vi "HFRR ADV v05 new software.vi"() -> ()   [LabVIEW 2025] (continued)
                "state1" <- w4567
              }
              frame Enabled {
              }
            }
            n3613 = stacked-sequence {
              tunnel: w4484 -> [w4592 _ _]
              tunnel: [_ _ w4608] -> _
              frame #0 {
                (unwired) FALSE ("convert eol (F)")
                w4594 = enum16{"start", "end", "current"}."start" ("pos mode (0:2)")
                n3614 = local read "Path"() -> (w4588:path)
                n3615 = Path To String(path=w4588) -> (string=w4600:string)
                n3616 = Concatenate Strings(w4600, "\\", "Sensor File Name") -> (w4601:string)
                n3617 = local write "standard output 2"(" ") -> ()
                n3618 = String To Path(string=w4601) -> (path=w4591:path)
                n3619 = call <vilib>:"Open_Create_Replace File.vi"("advisory dialog? (display:T)"=FALSE, "function (open:0)"=T25."create or replace", "file path"=w4591) -> ("error out"=w4604:errorcluster, "refnum"=w4603:refnum<file>)  [unwired: 5 in, 2 out]
                n3620 = Set File Position(refnum=w4603, from (0:start)=w4594, error in=w4604) -> (refnum out=w4584:refnum<file>, error out=w4583:errorcluster)  [unwired: 1 in]
                n3621 = Write to Binary File(file (use dialog)=w4584, data=" ", error in=w4583, 5:FALSE ("prepend array or string size? (T)")) -> (refnum out=w4595:refnum<file>, error out=w4596:errorcluster)  [unwired: 2 in, 1 out]
                n3622 = Set File Position(offset (in bytes) (0)=w4594, refnum=w4595, error in=w4596) -> (refnum out=w4587:refnum<file>, error out=w4586:errorcluster)  [unwired: 1 in]
                n3623 = Write to Binary File(file (use dialog)=w4587, data=w4592, error in=w4586, 5:FALSE ("prepend array or string size? (T)")) -> (error out=w4590:errorcluster)  [unwired: 2 in, 2 out]
                n3624 = flat-sequence {
                  tunnel: w4591 -> [w4606]
                  tunnel: w4590 -> [_]
                  frame #0 {
                    n3625 = call <vilib>:"Read Characters From File.vi"("file path (dialog if empty)"=w4606) -> ("character string"=→"Sensor Health JSON string":string)  [unwired: 5 in, 3 out]
                  }
                }
                "SinglePoint  2" <- w4592
              }
              frame #1 {
              }
              frame #2 {
                (unwired) "\"Stored\": true" ("string")
                n3626 = call <vilib>:"System Exec.vi"("run minimized? (F)"=TRUE, "wait until completion? (T)"=TRUE, "working directory"=path "C:/LAB-IQ-NXT", "command line"="C:\\LAB-IQ-NXT\\JPostH.bat") -> ("standard error"=→"Respose From Server 2":string, "standard output"=w4611:string)  [unwired: 4 in, 2 out]
                "standard output 2" <- w4611
                n3627 = Match Pattern(string=w4611, regular expression="JSONH Check String") -> (match substring=w4609:string, offset past match=w4608:i32)  [unwired: 1 in, 2 out]
                n3628 = Equal?(x=w4609, y="JSONH Check String") -> (x = y?=→"Upload \nConfirmed 2":bool)
              }
            }
            n3629 = Divide(x=w4451, y=3600.0 ("f")) -> (x/y=w4444:dbl)
            n3630 = local read "run time"() -> (w4501:string[])
            n3631 = Round To Nearest(number=w4444) -> (nearest integer value=w4443:dbl)
            n3632 = Number To Decimal String(number=w4443) -> (decimal integer string=w4442:string)  [unwired: 1 in]
            n3633 = Index Array(array="Sensor Information", index (col) #1=0 ("disabled index (col)"), index (col) #2=1 ("index (col)"), index (col) #3=2 ("index (col)"), index (col) #4=3 ("index (col)")) -> (element #1=→"Sensor name":string[], element #2=→"model num":string[], element #3=→"run time":string[], element #4=→"state":string[])  [unwired: 4 in]
            n3634 = Insert Into Array(array=w4501, index=1, new element #1=w4442, new element #2=w4442, new element #3=w4442, new element #4=w4442, new element #5=w4442, new element #6=w4442) -> (w4466:string[])
            "run" <- w4466
            n3635 = local read "out"() -> (w4448:string[])
            n3636 = local read "Sensor Information"() -> (w4468:string[][])
            n3637 = Replace Array Subset(array=w4468, new element #1=w4466, index (col) #1=2 ("disabled index (col)"), new element #2=w4448, index (col) #2=3 ("index (col)")) -> (w4467:string[][])  [unwired: 2 in]
            n3638 = local write "Sensor Information"(w4467) -> ()
          }
        }
        n3639 = case shown="True" w4415 {
          frame False {
          }
          frame True {
            n3640 = Equal?(x="FLAG", y=0.0) -> (x = y?=w4432:bool)
            n3641 = case shown="False" w4432 {
              frame False {
                n3642 = Get Date/Time In Seconds() -> (seconds since 1Jan1904=w4438:timestamp)
                n3643 = local read "START 2"() -> (w4436:dbl)
                n3644 = To Double Precision Float(number=w4438) -> (double precision float=w4437:dbl)
                n3645 = Subtract(x=w4437, y=w4436) -> (x-y=→"SENSOR TIME  2":dbl)
              }
              frame True {
                n3646 = Get Date/Time In Seconds() -> (seconds since 1Jan1904=w4440:timestamp)
                n3647 = To Double Precision Float(number=w4440) -> (double precision float=→"START 2":dbl)
                n3648 = local write "FLAG"(100.0 ("FLAG")) -> ()
              }
            }
          }
        }
        n3649 = disable-structure shown="Disabled" {
          disable-tunnel: w4418 -> [w4427 _]
          disable-tunnel: [w4426 _] -> w4417
          frame Disabled {
            n3650 = local read "Json St Flg"() -> (w4425:bool)
            n3651 = case shown="True" w4425 {
              tunnel: w4427 -> [w4428 w4430]
              tunnel: [w4428 w4429] -> w4426
              frame False {
              }
              frame True {
                n3652 = Increment(x=w4430) -> (x+1=w4429:dbl)
                "T cycle" <- w4429
                n3653 = local write "Json St Flg"(FALSE ("Json St Flg")) -> ()
              }
            }
          }
          frame Enabled {
          }
        }
        n3654 = local read "Quit"() -> (w4412:bool)
      }
    }
    frame Enabled {
    }
  }
  n3655 = stacked-sequence {
    tunnel: [w4810] -> w38
    frame #0 {
      w4810 = FALSE ("Upload \nConfirmed")
      n3656 = local write "Upload \nConfirmed"(w4810) -> ()
      n3657 = local write "St Str"("") -> ()
    }
  }
  n3658 = disable-structure shown="Disabled" {
    disable-tunnel: w38 -> [w4811 _]
    frame Disabled {
      n3659 = case shown="True" {
        selector: _ -> [_ _]
        tunnel: w4811 -> [_ w4812]
        frame False {
        }
        frame True {
          n3660 = while {
            tunnel: [w4818] -> _
            tunnel: w4812 -> [_]
            i -> [w4818]
            stop <- w4813 stop-if-true
            n3661 = local read "Json End Flg"() -> (w4817:bool)
            n3662 = Wait (ms)(milliseconds to wait=u32 20 ("Refresh Rate (ms)")) -> ()  [unwired: 1 out]
            n3663 = local read "refresh flag"() -> (w4814:bool)
            n3664 = local read "RUN"() -> (w4815:bool)
            n3665 = And(x=w4815, y=w4814) -> (x .and. y?=w4816:bool)
            n3666 = Or(x=w4816, y=w4817) -> (x .or. y?=w4819:bool)
            "AR Led" <- w4819
            n3667 = case shown="True" w4819 {
              frame False {
              }
              frame True {
                w4836 = "\",\""
                n3668 = local read "UUID"() -> (w4834:string)
                n3669 = local write "refresh flag"(FALSE ("refresh flag")) -> ()
                n3670 = local read "time"() -> (w4823:dbl)
                n3671 = Multiply(x=w4823, y=60.0) -> (x*y=w4822:dbl)
                n3672 = Concatenate Strings("UUID\" : \"", w4834, "\"}") -> (w4837:string)
                n3673 = Number To Fractional String(number=w4822, width (-)=i16 10, precision (6)=i16 4) -> (F-format string=w4851:string)  [unwired: 1 in]
                n3674 = Concatenate Strings("{", "\"Time\":\"", w4851, w4836) -> (w4846:string)
                n3675 = stacked-sequence {
                  tunnel: w4836 -> [w4899 w4907 w4914 w4922 w4930 w4939 w4946]
                  tunnel: [w4900 _ _ _ _ _ _] -> w4850
                  tunnel: [_ w4908 _ _ _ _ _] -> w4849
                  tunnel: [_ _ w4915 _ _ _ _] -> w4848
                  tunnel: [_ _ _ w4924 _ _ _] -> w4847
                  tunnel: w4837 -> [_ _ _ _ _ _ w4957]
                  tunnel: [_ _ _ _ _ _ w4956] -> w4833
                  tunnel: [_ _ _ _ _ w4936 _] -> w4832
                  tunnel: [_ _ _ _ w4929 _ _] -> w4831
                  frame #0 {
                    n3676 = local read "NORMAL LOAD"() -> (w4898:dbl)
                    n3677 = Number To Fractional String(number=w4898, width (-)=i16 10, precision (6)=i16 4) -> (F-format string=w4901:string)  [unwired: 1 in]
                    n3678 = Concatenate Strings("NormalLoad\":\"", w4901, w4899) -> (w4900:string)
                  }
                  frame #1 {
                    n3679 = local read "Temp"() -> (w4906:dbl)
                    n3680 = Number To Fractional String(number=w4906, width (-)=i16 10, precision (6)=i16 4) -> (F-format string=w4909:string)  [unwired: 1 in]
                    n3681 = Concatenate Strings("Temperature\":\"", w4909, w4907) -> (w4908:string)
                  }
                  frame #2 {
                    n3682 = local read "cof"() -> (w4912:dbl)
                    n3683 = Number To Fractional String(number=w4912, width (-)=i16 10, precision (6)=i16 4) -> (F-format string=w4916:string)  [unwired: 1 in]
                    n3684 = Concatenate Strings("FrictionalForce\":\"", w4916, w4914) -> (w4915:string)
                  }
                  frame #3 {
                    n3685 = local read "Set Hz"() -> (w4920:dbl)
                    n3686 = Multiply(x=w4920, y=60.0) -> (x*y=w4919:dbl)
                    n3687 = Number To Fractional String(number=w4919, width (-)=i16 10, precision (6)=i16 4) -> (F-format string=w4925:string)  [unwired: 1 in]
                    n3688 = Concatenate Strings("Speed\":\"", w4925, w4922) -> (w4924:string)
                  }
                  frame #4 {
                    n3689 = local read item#-1() -> (w4928)
                    n3690 = Number To Fractional String(number=w4928, width (-)=i16 10, precision (6)=i16 4) -> (F-format string=w4932:string)  [unwired: 1 in]
                    n3691 = Concatenate Strings("LinearDeformation\":\"", w4932, w4930) -> (w4929:string)
                  }
                  frame #5 {
                    n3692 = local read "AIR TEMP"() -> (w4935:dbl)
                    n3693 = local read "Json St Flg"() -> (w4937:bool)
                    n3694 = local read "Json End Flg"() -> (w4938:bool)
                    n3695 = Number To Fractional String(number=w4935, width (-)=i16 10, precision (6)=i16 4) -> (F-format string=w4941:string)  [unwired: 1 in]
                    n3696 = Concatenate Strings("Vibration\":\"", w4941, w4939) -> (w4936:string)
                    n3697 = And(x=w4937, y=w4938) -> ()  [unwired: 1 out]
                  }
                  frame #6 {
                    n3698 = local read "Json End Flg"() -> (w4945:bool)
                    n3699 = Get Date/Time In Seconds() -> (seconds since 1Jan1904=w4953:timestamp)
                    n3700 = local read "Json St Flg"() -> (w4944:bool)
                    n3701 = To Double Precision Float(number=w4953) -> (double precision float=w4952:dbl)
                    n3702 = Subtract(x=w4952, y=2082844800.0) -> (x-y=w4950:dbl)
                    n3703 = Number To Fractional String(number=w4950, width (-)=i16 12, precision (6)=i16 0) -> (F-format string=w4947:string)  [unwired: 1 in]
                    n3704 = case shown="True" w4945 {
                      tunnel: ["" w4960] -> w4954
                      tunnel: w4947 -> [_ w4961]
                      tunnel: w4946 -> [_ w4959]
                      frame False {
                      }
                      frame True {
                        n3705 = local write "Json End Flg"(FALSE ("Json St Flg")) -> ()
                        n3706 = Concatenate Strings("End\": \"", w4961, w4959) -> (w4960:string)
                      }
                    }
                    n3707 = case shown="True" w4944 {
                      tunnel: [w4964 w4967] -> w4955
                      tunnel: w4947 -> [_ w4968]
                      tunnel: w4946 -> [_ w4965]
                      frame False {
                        n3708 = local read "St Str"() -> (w4964:string)
                      }
                      frame True {
                        n3709 = Concatenate Strings("Start\":\"", w4968, w4965) -> (w4967:string)
                        "St Str" <- w4967
                        n3710 = local write "Json St Flg"(FALSE ("Json St Flg")) -> ()
                      }
                    }
                    n3711 = Concatenate Strings(w4955, w4954, w4957) -> (w4956:string)
                  }
                }
                n3712 = local read "FILE"() -> (w4825:string)
                n3713 = Concatenate Strings("\",\"OperatorID\":\"" ("string"), "Operator ID") -> (w4828:string)
                n3714 = Concatenate Strings("\",\"DatasetTitle\":\"" ("string"), w4825) -> (w4827:string)
                n3715 = Concatenate Strings("\",\"SerialNumber\":\"" ("string"), "Serial No") -> (w4857:string)
                n3716 = Concatenate Strings("\",\"ModelNumber\":\"" ("string"), "Model No") -> (w4856:string)
                n3717 = Concatenate Strings(w4857, w4856) -> (w4839:string)
                n3718 = Concatenate Strings("{\"SecretKey\":\"", "Secret Key", w4839, w4828, w4827, "\",\"Samples\":[") -> (w4844:string)
                n3719 = Concatenate Strings(w4846, w4850, w4849, w4848, w4847, w4831, w4832, w4833) -> (w4845:string)
                n3720 = Concatenate Strings(w4844, w4845, "]}") -> (w4843:string)
                n3721 = stacked-sequence {
                  tunnel: w4843 -> [w4872 _ _]
                  tunnel: [_ _ w4889] -> _
                  frame #0 {
                    (unwired) FALSE ("convert eol (F)")
                    w4874 = enum16{"start", "end", "current"}."start" ("pos mode (0:2)")
                    n3722 = Path To String(path="Path") -> (string=w4880:string)
                    n3723 = Concatenate Strings(w4880, "\\", "Data File Name") -> (w4882:string)
                    n3724 = local write "standard output"(" ") -> ()
                    n3725 = String To Path(string=w4882) -> (path=w4871:path)
                    n3726 = call <vilib>:"Open_Create_Replace File.vi"("advisory dialog? (display:T)"=FALSE, "function (open:0)"=T25."create or replace", "file path"=w4871) -> ("error out"=w4885:errorcluster, "refnum"=w4884:refnum<file>)  [unwired: 5 in, 2 out]
                    n3727 = Set File Position(refnum=w4884, from (0:start)=w4874, error in=w4885) -> (refnum out=w4865:refnum<file>, error out=w4864:errorcluster)  [unwired: 1 in]
                    n3728 = Write to Binary File(file (use dialog)=w4865, data=" ", error in=w4864, 5:FALSE ("prepend array or string size? (T)")) -> (refnum out=w4875:refnum<file>, error out=w4876:errorcluster)  [unwired: 2 in, 1 out]
                    n3729 = Set File Position(offset (in bytes) (0)=w4874, refnum=w4875, error in=w4876) -> (refnum out=w4868:refnum<file>, error out=w4867:errorcluster)  [unwired: 1 in]
                    n3730 = Write to Binary File(file (use dialog)=w4868, data=w4872, error in=w4867, 5:FALSE ("prepend array or string size? (T)")) -> (error out=w4870:errorcluster)  [unwired: 2 in, 2 out]
                    n3731 = flat-sequence {
                      tunnel: w4871 -> [w4887]
                      tunnel: w4870 -> [_]
                      frame #0 {
                        n3732 = call <vilib>:"Read Characters From File.vi"("file path (dialog if empty)"=w4887) -> ("character string"=→"JSON string":string)  [unwired: 5 in, 3 out]
                      }
                    }
                    "SinglePoint" <- w4872
                  }
                  frame #1 {
                  }
                  frame #2 {
                    (unwired) "\"Stored\": true" ("string")
                    n3733 = call <vilib>:"System Exec.vi"("run minimized? (F)"=TRUE, "wait until completion? (T)"=TRUE, "working directory"=path "C:/LAB-IQ-NXT", "command line"="C:\\LAB-IQ-NXT\\JPost.bat") -> ("standard error"=→"Respose From Server":string, "standard output"=w4892:string)  [unwired: 4 in, 2 out]
                    "standard output" <- w4892
                    n3734 = Match Pattern(string=w4892, regular expression="JSON Check String") -> (match substring=w4890:string, offset past match=w4889:i32)  [unwired: 1 in, 2 out]
                    n3735 = Equal?(x=w4890, y="JSON Check String") -> (x = y?=→"Upload \nConfirmed":bool)
                  }
                }
              }
            }
            n3736 = local read "Quit"() -> (w4813:bool)
          }
        }
      }
    }
    frame Enabled {
    }
  }
  n3737 = disable-structure shown="Disabled" {
    disable-tunnel: _ -> [w4975 _]
    frame Disabled {
      n3738 = while {
        shift-right: [w4983] -> w4971
        shift-left: _ -> [w4984]
        shift-right: [w4981] -> w4972
        shift-left: errorcluster {"status"=TRUE, "code"=0, "source"="Init"} ("error out") -> [w4982]
        shift-right: [w4979] -> _
        shift-left: "" -> [w4980]
        tunnel: [w4977] -> _
        tunnel: w4975 -> [_]
        i -> [w4977]
        stop <- w4976 stop-if-true
        n3739 = flat-sequence {
          tunnel: [w4985] -> w4978
          frame #0 {
            n3740 = Wait (ms)(milliseconds to wait=10.0 ("Delay")) -> (millisecond timer value=w4985:u32)
          }
        }
        n3741 = case shown="No Error" w4982 {
          selector: w4982 -> [w5015 w5134]
          tunnel: [w4998 w5136] -> w4983
          tunnel: [w4997 w5135] -> w4981
          tunnel: w4984 -> [w5016 w5128]
          tunnel: w4980 -> [w4996 w5127]
          tunnel: [w4995 w5127] -> w4979
          tunnel: w4978 -> [_ _]
          frame No Error {
            n3742 = Concatenate Strings("\r", "\n") -> (w5007:string)  [unwired: 1 in]
            n3743 = case shown="True" w5008 {
              tunnel: w5016 -> [w5040 w5047]
              tunnel: w5015 -> [w5039 w5046]
              tunnel: [w5040 w5045] -> w5014
              tunnel: [w5039 w5044] -> w4994
              tunnel: w5007 -> [_ w5043]
              frame False {
              }
              frame True {
                n3744 = VISA Write(VISA resource name=w5047, write buffer=w5043, error in (no error)=w5046) -> (VISA resource name out=w5045:refnum<visa-resource-name>, error out=w5044:errorcluster)  [unwired: 1 out]
                n3745 = local write "Read String"("") -> ()
                n3746 = local write item#-1(FALSE) -> ()
              }
            }
            n3747 = property class="Instr"(reference=w5014, error in=w4994) -> (reference out=w5013:refnum<visa-resource-name>, error out=w5012:errorcluster, "Serial Settings:Number of Bytes at Serial Port"=w5011:u32)
            n3748 = Greater?(x=w5011, y=u32 100) -> (0:w5009:bool)
            n3749 = case shown="True" w5009 {
              tunnel: w5013 -> [w5050 w5074]
              tunnel: w5012 -> [w5049 w5073]
              tunnel: w5011 -> [_ w5072]
              tunnel: [w5050 w5071] -> w5000
              tunnel: [w5049 w5070] -> w4999
              tunnel: w4996 -> [w5048 w5069]
              tunnel: [w5048 ""] -> w4995
              frame False {
              }
              frame True {
                w5059 = u32 6 ("y")
                # "Page 84 of \nmanual"
                n3750 = VISA Read(VISA resource name=w5074, byte count=w5072, error in (no error)=w5073) -> (VISA resource name out=w5071:refnum<visa-resource-name>, read buffer=w5067:string, error out=w5070:errorcluster)  [unwired: 1 out]
                n3751 = while {
                  tunnel: w5067 -> [w5123]
                  tunnel: [w5119] -> w5061 mode=indexing
                  tunnel: [w5113] -> w5065 mode=indexing
                  tunnel: [w5111] -> _
                  i -> [w5111]
                  stop <- w5116 stop-if-true
                  n3752 = String Subset(string=w5123, offset (0)=w5111) -> (substring=w5118:string)  [unwired: 1 in]
                  n3753 = String To Byte Array(string=w5118) -> (unsigned byte array=w5122:u8[])
                  n3754 = String Length(string=w5118) -> (length=w5117:i32)
                  n3755 = Index Array(array=w5122) -> (element=w5121:u8)  [unwired: 1 in]
                  n3756 = Equal To 0?(x=w5117) -> (x = 0?=w5116:bool)
                  n3757 = Number To Boolean Array(number=w5121) -> (Boolean array=w5115:bool[])
                  n3758 = Reverse 1D Array(array=w5115) -> (reversed array=w5114:bool[])
                  n3759 = And(x=w5115, y=bool[] [FALSE, FALSE, FALSE, FALSE, FALSE, FALSE, TRUE, TRUE] ("Boolean array")) -> (x .and. y?=w5119:bool[])
                  n3760 = And(x=w5114, y=bool[] [FALSE, FALSE, TRUE, TRUE, TRUE, TRUE, TRUE, TRUE] ("Boolean array")) -> (x .and. y?=w5113:bool[])
                }
                n3761 = Concatenate Strings(w5069, w5067) -> (→"Read String":string)
                n3762 = while {
                  tunnel: w5061 -> [w5110] mode=indexing
                  tunnel: [w5106] -> w5064
                  i -> [w5106]
                  stop <- w5107 stop-if-true
                  n3763 = Search 1D Array(1D array=w5110, element=TRUE) -> (index of element=w5108:i32)  [unwired: 1 in]
                  n3764 = Less Than 0?(x=w5108) -> (x < 0?=w5107:bool)
                }
                n3765 = Delete From Array(array=w5065, length=w5064, index (row)=0) -> (array with subset deleted=w5060:bool[][])  [unwired: 1 in, 1 out]
                n3766 = Array Size(array=w5060) -> (size(s)=w5062:i32[])
                n3767 = Index Array(array=w5062) -> (element=w5054:i32)  [unwired: 1 in]
                n3768 = Greater?(x=w5054, y=w5059) -> (0:w5057:bool)
                n3769 = Subtract(x=w5054, y=w5059) -> (x-y=w5058:u32)
                n3770 = Select(t=w5058, s=w5057, f=u32 0) -> (s? t:f=w5055:u32)
                n3771 = while {
                  tunnel: w5060 -> [w5093]
                  tunnel: [w5095] -> w5053 mode=indexing
                  tunnel: w5055 -> [w5077]
                  i -> [w5094]
                  stop <- w5092 stop-if-true
                  w5084 = 6 ("index")
                  w5083 = 2 ("length")
                  # "Page 65 of \nmanual"
                  n3772 = Multiply(x=u32 3 ("y"), y=w5094) -> (x*y=w5091:u32)
                  n3773 = Divide(x=u32 102 ("y"), y=u32 65520) -> (x/y=w5101:dbl)
                  n3774 = Greater Or Equal?(x=w5091, y=w5077) -> (x >= y?=w5092:bool)
                  n3775 = Index Array(array=w5093, index (row) #1=w5091) -> (element #1=w5089:bool[], element #2=w5088:bool[], element #3=w5087:bool[])  [unwired: 5 in]
                  n3776 = Reverse 1D Array(array=w5089) -> (reversed array=w5082:bool[])
                  n3777 = Reverse 1D Array(array=w5088) -> (reversed array=w5086:bool[])
                  n3778 = Reverse 1D Array(array=w5087) -> (reversed array=w5085:bool[])
                  n3779 = Delete From Array(array=w5082, length=w5083, index=w5084) -> (array with subset deleted=w5078:bool[])  [unwired: 1 out]
                  n3780 = Delete From Array(array=w5086, length=w5083, index=w5084) -> (array with subset deleted=w5079:bool[])  [unwired: 1 out]
                  n3781 = Delete From Array(array=w5085, length=w5083, index=w5084) -> (array with subset deleted=w5080:bool[])  [unwired: 1 out]
                  n3782 = Insert Into Array(array=bool[] [] ("Boolean array"), new element #1=w5078, new element #2=w5079, new element #3=w5080) -> (w5081:bool[])  [unwired: 1 in]
                  n3783 = Boolean Array To Number(Boolean array=w5081) -> (number=w5090:u32)
                  n3784 = Multiply(x=w5101, y=w5090) -> (x*y=w5100:dbl)
                  n3785 = Decrement(x=w5100) -> (x-1=w5099:dbl)
                  n3786 = Divide(x=w5099, y=u32 100) -> (x/y=w5097:dbl)
                  n3787 = Multiply(x=w5097, y=u32 10) -> (x*y=w5095:dbl)
                }
                n3788 = Delete From Array(array=w5053) -> (array with subset deleted=w5052:dbl[])  [unwired: 2 in, 1 out]
                "Waveform Graph 5" <- w5052
                "Waveform Chart 3" <- w5052
                n3789 = call-poly <vilib>:"Mean.vi"("X"=w5052) -> ("mean"=w5051:dbl)  [unwired: 1 out]
                n3790 = case shown="True" {
                  selector: _ -> [_ _]
                  tunnel: w5051 -> [_ w5076]
                  frame False {
                  }
                  frame True {
                    n3791 = local write item#-1(FALSE ("Zero 4")) -> ()
                    "z_measure" <- w5076
                  }
                }
              }
            }
            n3792 = local read item#-1() -> (w4991)
            n3793 = local read item#-1() -> (w4990)
            n3794 = local read item#-1() -> (w4992)
            n3795 = local read item#-1() -> (w4989)
            n3796 = case shown="True" w4987 {
              tunnel: w4991 -> [_ w5019]
              tunnel: w4992 -> [_ w5018]
              frame False {
              }
              frame True {
                n3797 = Build Array(w5019, w5018) -> (w5017:void[])
                n3798 = local read item#-1() -> (w5022)
                n3799 = Build Array (concatenate)(w5022, w5017) -> (w5020:void[])
                n3800 = local write item#-1(w5020) -> ()
                n3801 = local write item#-1(FALSE ("Boolean 8")) -> ()
              }
            }
            n3802 = call "Build XY Graph"("Enable"=w4989, "Reset"=w4990, "Y Input"=w4992, "X Input"=w4991) -> ("XY Graph"=w4988:cluster{"Y":dbl[], "Y":dbl[]}[])  [unwired: 6 in, 1 out]
            n3803 = case shown="True" {
              selector: _ -> [_ _]
              frame False {
              }
              frame True {
                n3804 = local read item#-1() -> (w5023)
                n3805 = Index Array(array=w5023, index (col) #1=0 ("disabled index (col)"), index (col) #2=1 ("index (col)")) -> (element #1=w5025, element #2=w5024)  [unwired: 2 in]
                n3806 = call <vilib>:"Linear Fit.vi"("Y"=w5025, "X"=w5024) -> ()  [unwired: 9 in, 5 out]
                n3807 = local write item#-1(FALSE ("Boolean 9")) -> ()
              }
            }
            n3808 = case shown="True" {
              selector: _ -> [_ _]
              frame False {
              }
              frame True {
                n3809 = local write item#-1(dbl[][] [] ("Captured Values")) -> ()
                n3810 = local write item#-1(FALSE ("Boolean 7")) -> ()
              }
            }
            n3811 = Concatenate Strings("\r", "\n") -> (w5002:string, w5001:string)
            n3812 = case shown="True" w4993 {
              tunnel: w5000 -> [w5032 w5038]
              tunnel: w4999 -> [w5031 w5037]
              tunnel: [w5032 w5036] -> w4998
              tunnel: [w5031 w5035] -> w4997
              tunnel: w5002 -> [_ w5034]
              frame False {
              }
              frame True {
                n3813 = VISA Write(VISA resource name=w5038, write buffer=w5034, error in (no error)=w5037) -> (VISA resource name out=w5036:refnum<visa-resource-name>, error out=w5035:errorcluster)  [unwired: 1 out]
                n3814 = local write item#-1(FALSE ("WRITE")) -> ()
              }
            }
          }
          frame Error {
            w5126 = u16 10 items=["1.0"=10, "1.5"=15, "2.0"=20] ("stop bits (10: 1 bit)")
            n3815 = Wait (ms)(milliseconds to wait=u32 20) -> ()  [unwired: 1 out]
            n3816 = VISA Close(VISA resource name=w5128, error in (no error)=w5134) -> (error out=w5133:errorcluster)
            n3817 = call <vilib>:"Clear Errors.vi"("error in (no error)"=w5133) -> ("error out"=w5132:errorcluster)  [unwired: 5 in, 1 out]
            n3818 = call-poly "VISA Configure Serial Port"("timeout (10sec)"=u32 200, "Enable Termination\nChar (T)"=TRUE ("Enable Termination\nChar (T)"), "baud rate (9600)"=u32 921600, "error in (no error)"=w5132, "stop bits (10: 1 bit)"=w5126) -> ("VISA resource name"=w5124:refnum<visa-resource-name>, "VISA resource name out"=w5136:refnum<visa-resource-name>, "error out"=w5135:errorcluster)  [unwired: 8 in]
          }
        }
        n3819 = local read "Quit"() -> (w4976:bool)
      }
      n3820 = VISA Close(VISA resource name=w4971, error in (no error)=w4972) -> (error out=w4970:errorcluster)
      n3821 = call <vilib>:"Clear Errors.vi"("error in (no error)"=w4970) -> ()  [unwired: 5 in, 2 out]
    }
    frame Enabled {
    }
  }
  n3822 = disable-structure shown="Disabled" {
    disable-tunnel: _ -> [w5141 _]
    frame Disabled {
      n3823 = while {
        tunnel: [w5148] -> _
        shift-right: [w5145] -> w5138
        shift-left: _ -> [w5147]
        shift-right: [w5146] -> w5139
        shift-left: errorcluster {"status"=TRUE, "code"=0, "source"="Init"} ("error out") -> [w5144]
        tunnel: w5141 -> [_]
        i -> [w5148]
        stop <- w5142 stop-if-true
        n3824 = flat-sequence {
          tunnel: w5144 -> [w5239]
          tunnel: [w5239] -> w5143
          frame #0 {
            n3825 = Wait (ms)(milliseconds to wait=u32 50) -> ()  [unwired: 1 out]
          }
        }
        n3826 = case shown="No Error" w5143 {
          selector: w5143 -> [w5189 w5232]
          tunnel: w5147 -> [w5188 w5231]
          tunnel: [w5155 w5222] -> w5146
          tunnel: [w5156 w5230] -> w5145
          frame No Error {
            w5182 = T26 {"Mode"=enum."RTU", "Slave Address"=1} ("Serial Parameters")
            n3827 = call-poly <vilib>:"MB Serial Master Query (poly).vi"("VISA resource name"=w5188, "Starting Address"=i16 1000, "Quantity"=u16 1, "Timeout"=u32 1000, "error in"=w5189, "Serial Parameters"=w5182) -> ("VISA resource name out"=w5183:refnum<visa-resource-name>, "Input Registers"=w5185:u16[], "error out"=w5181:errorcluster)  [unwired: 10 in, 1 out]
            n3828 = Random Number (0-1)() -> (number: 0 to 1=w5170:dbl)
            n3829 = Index Array(array=w5185, index=0) -> (element=w5180:u16)
            n3830 = Subtract(x=w5170, y=0.5) -> (x-y=w5169:dbl)
            n3831 = Divide(x=w5180, y=10 ("index")) -> (x/y=w5174:dbl)
            n3832 = Multiply(x=w5169, y=0.5) -> (x*y=w5168:dbl)
            n3833 = Add(x=w5174, y=w5168) -> (x+y=w5173:dbl)
            n3834 = local read "Amb temp"() -> (w5157:dbl)
            n3835 = Multiply(x=w5173, y=0.2) -> (x*y=w5177:dbl)
            n3836 = Multiply(x=w5157, y=0.8) -> (x*y=w5175:dbl)
            n3837 = Add(x=w5177, y=w5175) -> (x+y=w5158:dbl)
            n3838 = local read "set temp old"() -> (w5152:dbl)
            n3839 = local write "Amb temp"(w5158) -> ()
            n3840 = Select(t="SetTemp 2", s="Heater", f=100.0) -> (s? t:f=w5153:dbl)
            n3841 = Not Equal?(x=w5153, y=w5152) -> (x != y?=w5151:bool)
            n3842 = case shown="True" w5151 {
              tunnel: w5183 -> [w5217 w5219]
              tunnel: [w5216 w5219] -> w5163
              tunnel: w5181 -> [w5215 w5218]
              tunnel: [w5214 w5218] -> w5161
              tunnel: w5153 -> [w5209 _]
              tunnel: w5182 -> [w5211 w5220]
              tunnel: [w5211 w5220] -> w5164
              frame True {
                n3843 = Multiply(x=w5209, y=10 ("index")) -> (x*y=w5208:dbl)
                n3844 = call-poly <vilib>:"MB Serial Master Query (poly).vi"("VISA resource name"=w5217, "Address"=u16 0, "Holding Register"=w5208, "Timeout"=u32 1000, "error in"=w5215, "Serial Parameters"=w5211) -> ("VISA resource name out"=w5216:refnum<visa-resource-name>, "error out"=w5214:errorcluster)  [unwired: 11 in, 1 out]
                "set temp old" <- w5209
              }
              frame False {
              }
            }
            n3845 = flat-sequence {
              tunnel: [w5190] -> _
              tunnel: [w5190] -> w5160
              tunnel: w5161 -> [w5190]
              frame #0 {
                n3846 = Wait (ms)(milliseconds to wait=u32 100) -> ()  [unwired: 1 out]
              }
            }
            n3847 = call "Elapsed Time12"("Time Target (s)"=2.0, "Auto Reset"=TRUE) -> ("Time has Elapsed"=w5165:bool)  [unwired: 10 in, 7 out]
            n3848 = case shown="True" w5165 {
              tunnel: w5164 -> [w5194 w5207]
              tunnel: [w5194 w5207] -> _
              tunnel: [w5193 w5205] -> w5156
              tunnel: w5163 -> [w5193 w5206]
              tunnel: [w5192 w5203] -> w5155
              tunnel: w5160 -> [w5192 w5204]
              frame False {
              }
              frame True {
                n3849 = call-poly <vilib>:"MB Serial Master Query (poly).vi"("VISA resource name"=w5206, "Starting Address"=i16 1003 ("Addr"), "Quantity"=u16 1, "Timeout"=u32 1000, "error in"=w5204, "Serial Parameters"=w5207) -> ("VISA resource name out"=w5205:refnum<visa-resource-name>, "Input Registers"=w5200:u16[], "error out"=w5203:errorcluster)  [unwired: 10 in, 1 out]
                n3850 = Index Array(array=w5200, index=0) -> (element=w5199:u16)
                n3851 = Divide(x=w5199, y=u16 10) -> (x/y=w5195:dbl)
                n3852 = local write "set temp old"(w5195) -> ()
                n3853 = local write "SetTemp"(w5195) -> ()
              }
            }
            "Error Code" <- w5155
            n3854 = Unbundle(w5155) -> ("status"=→"TK4 status":bool)  [unwired: 2 out]
            "SetTemp" <- "SetTemp 2"
          }
          frame Error {
            w5234 = u16 0 items=["None", "Odd", "Even", "Mark", "Space"] ("Parity")
            w5235 = u16 0 items=["None", "XON/XOFF", "RTS/CTS", "XON/XOFF & RTS/CTS", "DTR/DSR", "XON/XOFF & DTR/DSR"] ("Flow Control")
            n3855 = VISA Clear(VISA resource name=w5231, error in (no error)=w5232) -> (VISA resource name out=w5225:refnum<visa-resource-name>, error out=w5223:errorcluster)
            n3856 = VISA Close(VISA resource name=w5225, error in (no error)=w5223) -> (error out=w5224:errorcluster)
            n3857 = call <vilib>:"Clear Errors.vi"("error in (no error)"=w5224) -> ("error out"=w5233:errorcluster)  [unwired: 5 in, 1 out]
            n3858 = Unbundle By Name(T26 {"Mode"=enum."RTU", "Slave Address"=1} ("input cluster")) -> ("Mode"=w5236:enum16{"RTU", "ASCII"})
            n3859 = call <vilib>:"MB Serial Init.vi"("Timeout"=u32 100, "Flow Control"=w5235, "Mode"=w5236, "error in (no error)"=w5233, "Parity"=w5234, "Baud Rate"=u32 9600, "VISA resource name"="Lubrication System COM Port :") -> ("error out"=w5222:errorcluster, "VISA resource name out"=w5230:refnum<visa-resource-name>)  [unwired: 3 in]
            n3860 = local write "set temp old"(0.0 ("set temp old")) -> ()
            n3861 = Unbundle(w5222) -> ("status"=w5221:bool)  [unwired: 2 out]
            n3862 = case shown="True" w5221 {
              selector: w5221 -> [_ w5238]
              frame False {
              }
              frame True {
                n3863 = local write "TK4 status"(w5238) -> ()
              }
            }
          }
        }
        n3864 = local read "Quit"() -> (w5142:bool)
      }
      n3865 = VISA Close(VISA resource name=w5138, error in (no error)=w5139) -> (error out=w5137:errorcluster)
      n3866 = call <vilib>:"Clear Errors.vi"("error in (no error)"=w5137) -> ()  [unwired: 5 in, 2 out]
    }
    frame Enabled {
    }
  }
